vi "Link.vi"(0 "Timeout in":refnum<class "Timeout.lvclass">, 7 "State names":string[](array[string]), 11 "error in (no error)":errorcluster) -> (4 "Timeout out":refnum<class "Timeout.lvclass">, 15 "error out":errorcluster)   [LabVIEW 2020, in "Timeout.lvclass"]
uses:
  Timeout.lvclass
  Timeout.lvclass/Timeout.ctl
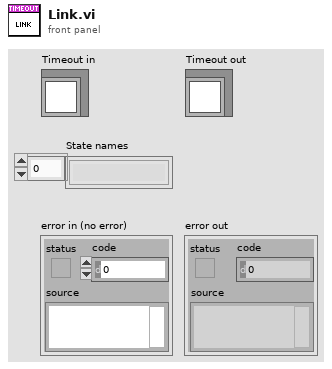
[diagram p1: front panel]
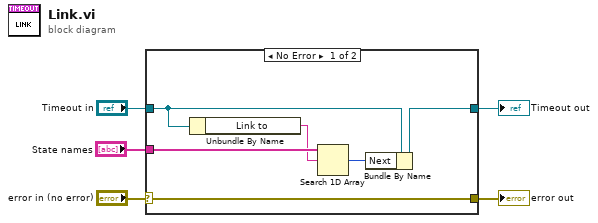
[diagram p0: block diagram]
diagram:
  n1 = case shown="No Error" "error in (no error)" {
    selector: "error in (no error)" -> [w11 w13]
    tunnel: [w11 w13] -> w4
    tunnel: [w10 w12] -> w2
    tunnel: "Timeout in" -> [w9 w12]
    tunnel: "State names" -> [w8 _]
    frame No Error {
      n2 = Unbundle By Name(w9) -> ("Link to"=w7:string)
      n3 = Search 1D Array(1D array=w8, element=w7) -> (index of element=w6:i32)  [unwired: 1 in]
      n4 = Bundle By Name(cluster=w9, "Next"=w6) -> (w10:refnum<class "Timeout.lvclass">)
    }
    frame Error {
    }
  }
  "error out" <- w4
  "Timeout out" <- w2
